vi "Ctor.vi"(8 "error in (no error)":errorcluster) -> (0 "error out":errorcluster, 3 "Timer Demo App out":refnum<class "Timer Demo App.lvclass">)   [LabVIEW 2020, in "Timer Demo.lvlib" / "Timer Demo App.lvclass"]
uses:
  Timer Demo App.lvclass
  Timer Demo App.lvclass/Timer Demo App.ctl
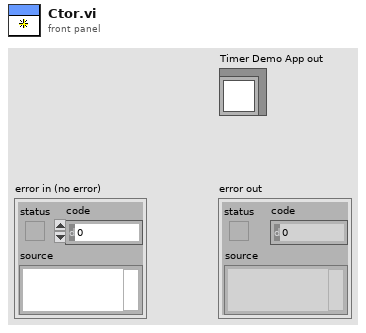
[diagram p1: front panel]
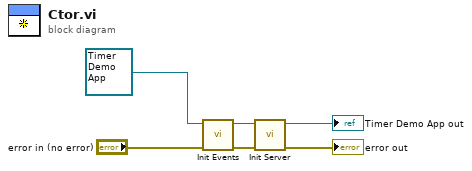
[diagram p0: block diagram]
diagram:
  n1 = call "Init Events.vi"("error in (no error)"="error in (no error)", "Timer Demo App in"=refnum<class "Timer Demo App.lvclass"> refnum) -> ("error out"=w3:errorcluster, "Timer Demo App out"=w4:refnum<class "Timer Demo App.lvclass">)  [unwired: 8 in]
  n2 = call "Init Server.vi"("error in (no error)"=w3, "Timer Demo App in"=w4) -> ("error out"=→"error out":errorcluster, "Timer Demo App out"=→"Timer Demo App out":refnum<class "Timer Demo App.lvclass">)  [unwired: 8 in]
